vi "TcXxx-xxx_Template.vi"(1 "Input buffer":T3="1", 3 "Invocation info":T2, 5 "error in (no error)":errorcluster, 6 "Add log to result?":bool) -> (16 "Test Data":T1 {"Numeric Measurement" format="%.2f"}, 19 "error out":errorcluster)   [LabVIEW 2009]
doc: "Test case template."
uses:
  Shared/Support_InputBuffer.ctl
  Shared/Support_InvocationInfo.ctl
  Shared/Support_TestData.ctl
panel:
  in  "Test name":string="TcXxx-xxx Template"
  out "Test result":bool
  out "Result":string
  # "Test case purpose..."
  # "Sub test case"
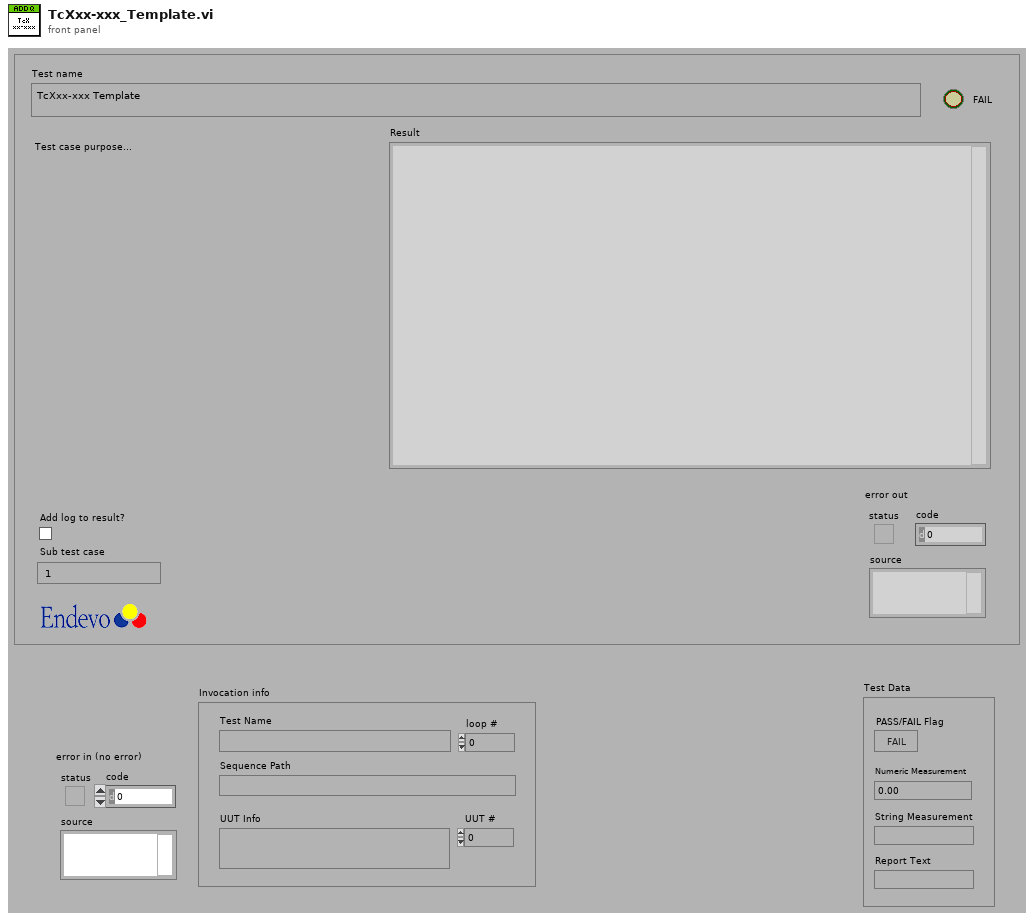
[diagram p1: front panel]
types:
  T1 = typedef "Support_TestData.ctl" = cluster{"PASS/FAIL Flag":bool, "Numeric Measurement":dbl, "String Measurement":string, "Report Text":string}
  T2 = typedef "Support_InvocationInfo.ctl" = cluster{"UUT #":i32, "loop #":i32, "UUT Info":string, "Test Name":string, "Sequence Path":path}
  T3 = typedef "Support_InputBuffer.ctl" = string
  T4 = typedef "Support_ResultType.ctl" = cluster{"Pass":bool, "Comment":string, "MeasurementValue":dbl}
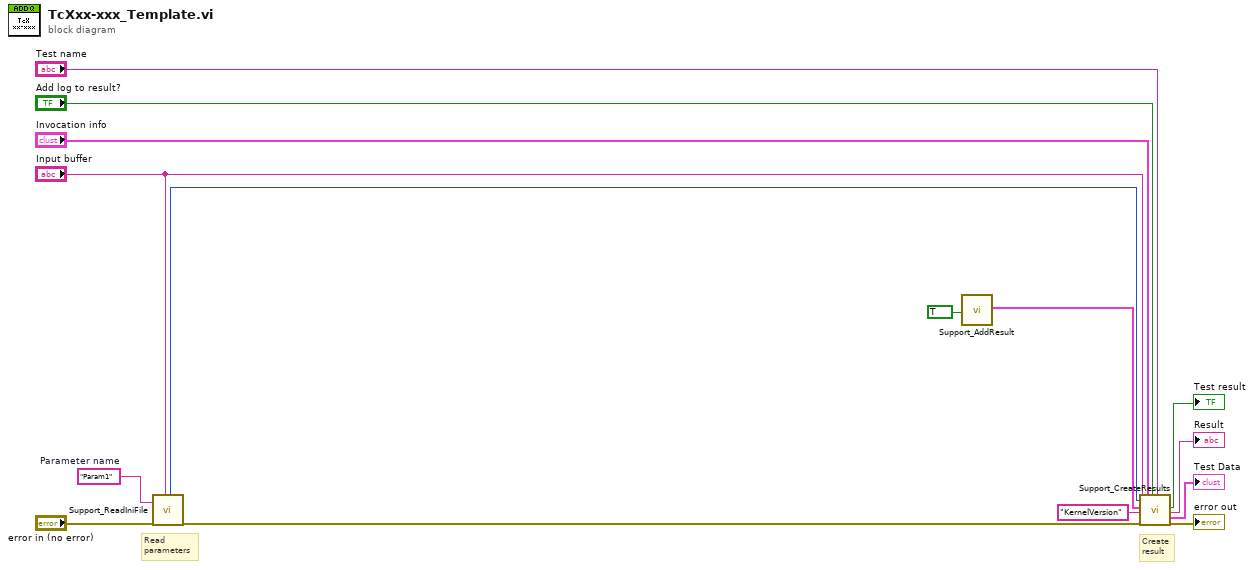
[diagram p0: block diagram]
diagram:
  w8 = "Param1"  # Parameter name
  # "Create\nresult"
  # "Read\nparameters"
  n1 = call "Support_ReadIniFile.vi"("Parameter name"=w8, "error in (no error)"="error in (no error)", "Sub test case"="Input buffer") -> ("Timer start"=w1:u32, "error out"=w10:errorcluster)  [unwired: 9 in, 6 out]
  n2 = call "Support_AddResult.vi"("Pass"=TRUE) -> ("Results out"=w6:T4[])  [unwired: 18 in]
  n3 = call "Support_CreateResults.vi"("Sub test case"="Input buffer", "Timer start"=w1, "Results"=w6, 3:"KernelVersion" ("Kernel version"), "error in (no error)"=w10, "Invocation info"="Invocation info", "Add log to result?"="Add log to result?", "Test name"="Test name") -> ("Pass/fail flag"=→"Test result":bool, "Result"=→"Result":string, "Test Data"=→"Test Data":T1, "error out"=→"error out":errorcluster)  [unwired: 8 in]
